vi "Tester.vi"() -> ()   [LabVIEW 2012]
uses:
  <vilib>/Platform/TimedLoop/XDataNode/timing_clust.ctl
  <vilib>/Platform/TimedLoop/XDataNode/nitl_modes.ctl
  <vilib>/Platform/TimedLoop/XDataNode/wakeup.ctl
  <vilib>/rvi/Emulation/niFpgaSctlEmulationRegisterWithScheduler.vi
  <vilib>/rvi/eio/common/nirviEmuTemplateMethod_errors.vi
  <vilib>/rvi/Emulation/niFpgaSctlEmulationScheduler.vi
  <vilib>/rvi/FIFO/Fifo_Resource/nirvififoEmulationSetSize.vi
  <vilib>/rvi/DataTransferAndStorage/Container/Common/niFpgaContainerGetUniqueNameForEmu.vi
  <vilib>/rvi/errors/niFpgaSetErrorForExecOnDevCompSimple.vi
  <vilib>/rvi/eio/common/nirviEmuReportErrorAndStop.vi
  <vilib>/rvi/Emulation/niFpgaSctlEmulationFifoFullMgr.vi
  <vilib>/rvi/Emulation/niFpgaSctlEmulationResourceMgr.vi
  <vilib>/rvi/interface/RandomDataEmulation/nirviRandomDataFPGAFIFO.vi
  <vilib>/rvi/interface/RandomDataEmulation/niFpgaRandomDataHandleErrors.vi
  <vilib>/rvi/Emulation/niFpgaSctlEmulationGlobalWrite.vi
  <vilib>/Platform/TimedLoop/XDataNode/XDataNode.xnode
  <vilib>/eio/EIONode/EIONode.xnode
  <vilib>/rvi/DataTransferAndStorage/Container/XNode/niFpgaContainer.xnode
  <vilib>/rvi/FIFO/Fifo_Resource/nirvififoEmulationClear.vi
  <vilib>/rvi/FIFO/Fifo_Resource/nirvififoEmulationWrite.vi
  <vilib>/rvi/FIFO/Fifo_Resource/nirvififoEmulationRead.vi
  <vilib>/rvi/interface/RandomDataEmulation/nirviRandomDataFpgaReadWriteTemplate.vi
  <vilib>/Platform/TimedLoop/XDataNode/XDNodeRunTimeDep.lvlib
panel:
  out "ToHostArea1LaserRaw FIFO Overflow":bool
  out "ToHostAreas FIFO Overflow":bool
  in  "Laser bitslip":bool
  in  "Laser delay inc":bool
  out "ToHost FIFO Overflow A2Ch1":bool
  in  "Samples per pixel Acq A2":u16=10000 caption="Samples per pixel Acq"
  in  "Samples per pixel Acq A1":u16=10000 caption="Samples per pixel Acq"
  in  "Requested pixels A2":u32=100000 caption="Requested pixels"
  in  "Samples per pixel A2":u16=10000 caption="Samples per pixel"
  out "ToHost FIFO Overflow A1Ch1":bool
  out "Acquiring":bool
  in  "Wait for trigger":bool
  in  "Acquire continuously":bool=TRUE
  in  "Requested pixels A1":u32=100000 caption="Requested pixels"
  in  "Clear Interloop FIFO":bool
  out "Interloop FIFO overflow":bool
  in  "Samples per pixel A1":u16=10000 caption="Samples per pixel"
  in  "Acquire":bool
  out "Interloop FIFO timeout":bool
  in  "Commit":bool
  out "Xpoint_Switch_Ready":bool
  in  "Xpoint_Switch_Write":bool
  in  "Clock Source":u8(ring)=3 items=["Tristate"=0, "Sync Clock (PXIe only)"=2, "Adapter Module Onboard Clock"=3, "Strobe from Crosspoint Switch"=4, "Strobe Bypass"=5]
  in  "Onboard_Clock_Write":bool
  in  "Onboard_Clock_Write_Data":u16
  out "Onboard_Clock_Ready":bool
  in  "Acq_Reset":bool
  # "6587 IO module configuration"
  # "Tester"
  # "Acquisition control"
  # "Area 1"
  # "Area 2"
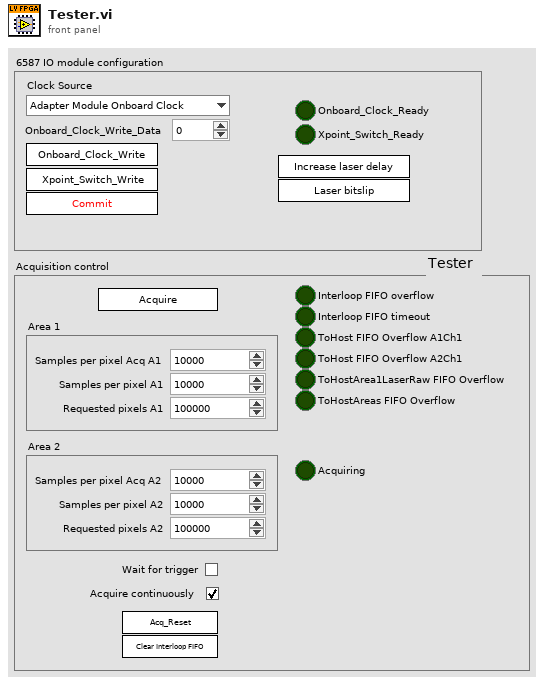
[diagram p1: front panel]
types:
  T1 = typedef "XDNodeRunTimeDep.lvlib/timing_clust.ctl" = cluster{"Expected End [f-1]":u64, "Actual End [f-1]":u64, "Finished Late? [f-1]":bool, "Expected End [i-1]":u64, "Actual End [i-1]":u64, "Finished Late? [i-1]":bool, "Expected Start [i]":u64, "Actual Start [i]":u64, "Expected Start [f]":u64, "Actual Start [f]":u64, "Source Name":string, "Structure Name":string, "Period":i64, "Deadline":i64, "Offset":i64, "Start":i64, "Priority":i32, "Timeout":i32, "Mode":T2, "Wakeup Reason":T3, "Error":errorcluster, "Source Type":string, "Secondary Source Type":string, "Global End Time":u64, "Global Start Time":u64, "Frame Duration":u64, "Iteration Duration":u64, "Assigned CPU":i32, "I/O Scan Engine Mode":u32}
  T2 = typedef "XDNodeRunTimeDep.lvlib/nitl_modes.ctl" = enum32{"No Change", "Process missed periods, maintain original phase", "Discard missed periods, maintain original phase", "Process missed periods, ignore original phase", "Discard missed periods, ignore original phase"}
  T3 = typedef "XDNodeRunTimeDep.lvlib/wakeup.ctl" = enum32{"Normal", "Aborted", "Asynchronous wakeup", "Timing source error", "Timed loop error", "Timeout"}
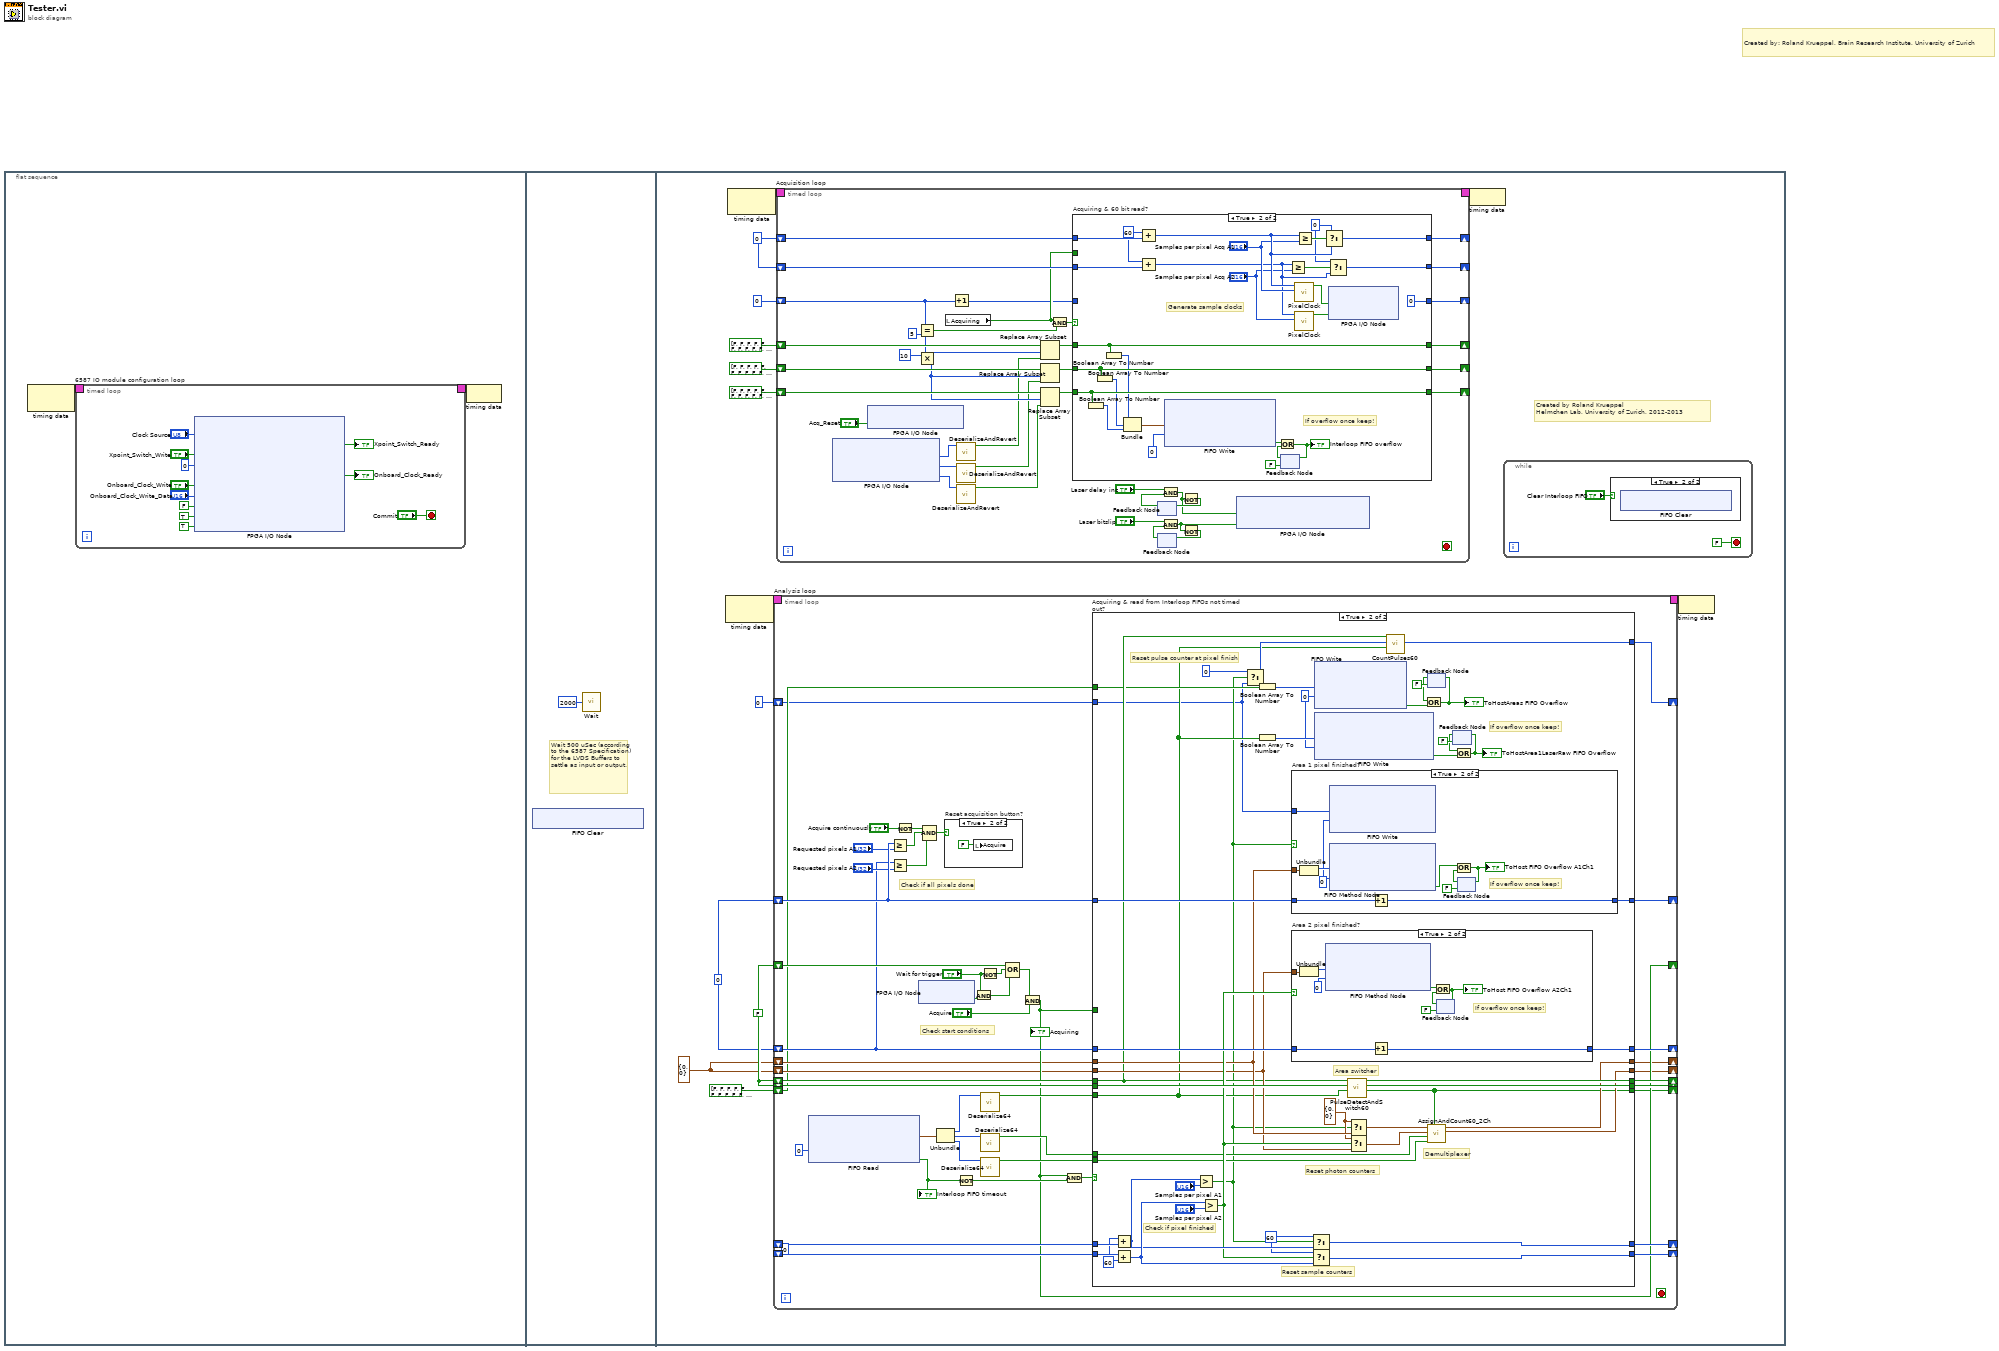
[diagram p0: block diagram]
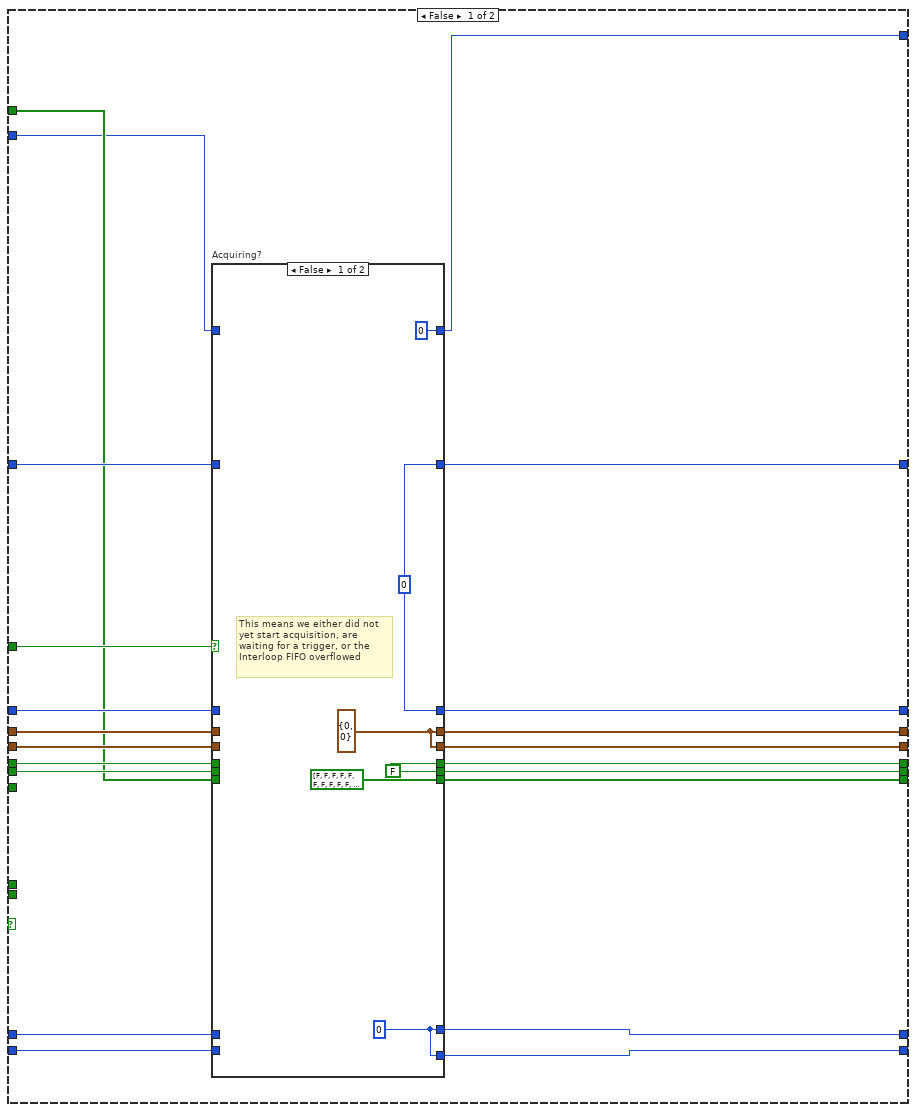
[diagram p4: hidden frame]
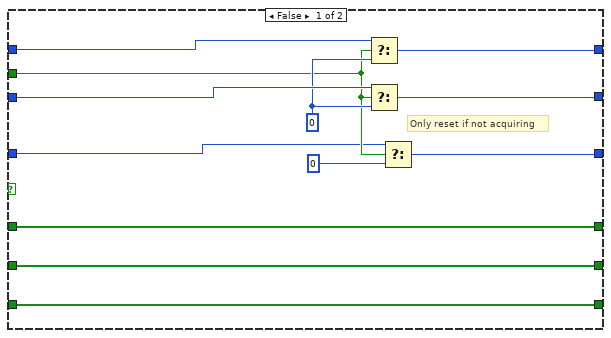
[diagram p8: hidden frame]
diagram:
  # "Created by: Roland Krueppel, Brain Research Institute, University of Zurich"
  n1 = flat-sequence {
    frame #0 {
      n2 = node-c288() -> (w2:T1)  [unwired: 1 in]
      n3 = timed-loop "6587 IO module configuration loop" {
        timing: w2 -> [_]
        timing-out: [_] -> w1
        stop <- "Commit" stop-if-true
        n4 = xnode "FPGA I/O Node"("IO Module\\Acq_IO_Clock_Source"="Clock Source", "IO Module\\Xpoint_Switch_Write"="Xpoint_Switch_Write", "IO Module\\LVDS_Data_Dir"=u16 0 ("IO Module\\LVDS_Data_Dir"), "IO Module\\Onboard_Clock_Write"="Onboard_Clock_Write", "IO Module\\Onboard_Clock_Write_Data"="Onboard_Clock_Write_Data", "IO Module\\SE_PFI0_WE"=FALSE ("IO Module\\SE_PFI0_WE"), "IO Module\\SE_PFI1_WE"=TRUE ("IO Module\\SE_PFI1_WE"), "IO Module\\SE_PFI2_WE"=TRUE ("IO Module\\SE_PFI2_WE")) -> ("IO Module\\Xpoint_Switch_Ready"=→"Xpoint_Switch_Ready":bool, "IO Module\\Onboard_Clock_Ready"=→"Onboard_Clock_Ready":bool)  [unwired: 10 in, 10 out]
      }
      n5 = node-c288(w1) -> ()
    }
    frame #1 {
      # "Wait 500 uSec (according to the 6587 Specification) for the LVDS Buffers to settle as input or output."
      n6 = xnode "FIFO Clear"() -> ()  [unwired: 1 in, 1 out]
      n7 = call "Wait"("Count(uSec)"=u32 2000) -> ()  [unwired: 1 out]
    }
    frame #2 {
      w21 = cluster{u16, u16} {0, 0} ("output cluster")
      w22 = u16 0
      w23 = u32 0 ("Cycle counter out")
      w24 = u16 0
      w25 = FALSE ("Last laser bit out")
      # "Created by Roland Krueppel\nHelmchen Lab, University of Zurich, 2012-2013"
      n8 = node-c288() -> (w31:T1)  [unwired: 1 in]
      n9 = node-c288() -> (w33:T1)  [unwired: 1 in]
      n10 = timed-loop "Analysis loop" {
        timing: w31 -> [_]
        timing-out: [_] -> w30
        shift-right: [w78] -> _
        shift-left: w25 -> [w81]
        shift-right: [w80] -> _
        shift-left: w25 -> [w79]
        shift-right: [w54] -> _
        shift-left: w24 -> [w77]
        shift-right: [w52] -> _
        shift-left: w23 -> [w76]
        shift-right: [w50] -> _
        shift-left: w25 -> [w65]
        shift-right: [w53] -> _
        shift-left: w24 -> [w60]
        shift-right: [w51] -> _
        shift-left: w23 -> [w58]
        shift-right: [w41] -> _
        shift-left: w21 -> [w43]
        shift-right: [w40] -> _
        shift-left: w21 -> [w42]
        shift-right: [w39] -> _
        shift-left: bool[] [FALSE, FALSE, FALSE, FALSE, FALSE, FALSE, FALSE, FALSE, FALSE, FALSE, FALSE, FALSE, FALSE, FALSE, FALSE, FALSE, FALSE, FALSE, FALSE, FALSE, FALSE, FALSE, FALSE, FALSE, FALSE, FALSE, FALSE, FALSE, FALSE, FALSE, FALSE, FALSE, FALSE, FALSE, FALSE, FALSE, FALSE, FALSE, FALSE, FALSE, FALSE, FALSE, FALSE, FALSE, FALSE, FALSE, FALSE, FALSE, FALSE, FALSE, FALSE, FALSE, FALSE, FALSE, FALSE, FALSE, FALSE, FALSE, FALSE, FALSE] ("Area bits out") -> [w38]
        shift-right: [w37] -> _
        shift-left: u16 0 ("New pulse count") -> [w36]
        stop <- _ stop-if-true
        # "Check start conditions"
        # "Check if all pixels done"
        n11 = xnode ("FIFO Read")("Timeout"=0) -> ("Element"=w47:cluster{"Laser":u64, "Ch0":u64, "Ch1":u64}, "Timed Out?"=w48:bool)  [unwired: 1 in, 1 out]
        "Interloop FIFO timeout" <- w48
        n12 = Greater Or Equal?(x=w76, y="Requested pixels A1") -> (x >= y?=w56:bool)
        n13 = Greater Or Equal?(x=w58, y="Requested pixels A2") -> (x >= y?=w55:bool)
        n14 = Not(x="Acquire continuously") -> (.not. x?=w57:bool)
        n15 = xnode "FPGA I/O Node"() -> ("TriggerIn"=w71:bool)  [unwired: 1 in, 1 out]
        n16 = Compound Arithmetic op=AND(w57, w56, w55) -> (w73:bool)
        n17 = Unbundle(w47) -> ("Laser"=w46:u64, "Ch0"=w45:u64, "Ch1"=w44:u64)
        n18 = case "Reset acquisition button?" shown="True" w73 {
          frame False {
          }
          frame True {
            n19 = local write "Acquire"(FALSE ("Acquire")) -> ()
          }
        }
        n20 = Not(x=w48) -> (.not. x?=w66:bool)
        n21 = And(x="Wait for trigger", y=w71) -> (x .and. y?=w68:bool)
        n22 = call "Deserialize64.vi"("U64 input"=w46) -> ("60bit output"=w63:bool[])  [unwired: 10 in]
        n23 = call "Deserialize64.vi"("U64 input"=w45) -> ("60bit output"=w62:bool[])  [unwired: 10 in]
        n24 = call "Deserialize64.vi"("U64 input"=w44) -> ("60bit output"=w61:bool[])  [unwired: 10 in]
        n25 = Not(x="Wait for trigger") -> (.not. x?=w69:bool)
        n26 = Compound Arithmetic op=OR(w65, w69, w68) -> (w67:bool)
        n27 = And(x=w67, y="Acquire") -> (x .and. y?=w50:bool)
        "Acquiring" <- w50
        n28 = And(x=w50, y=w66) -> (x .and. y?=w64:bool)
        n29 = case "Acquiring & read from Interloop FIFOs not timed out?" shown="True" w64 {
          tunnel: w81 -> [w98 w152]
          tunnel: w43 -> [w102 w148]
          tunnel: [w97 w151] -> w80
          tunnel: w79 -> [w99 w138]
          tunnel: [w96 w150] -> w78
          tunnel: w77 -> [w101 w166]
          tunnel: w76 -> [w100 w162]
          tunnel: w63 -> [_ w131]
          tunnel: w62 -> [_ w144]
          tunnel: w50 -> [w103 _]
          tunnel: w61 -> [_ w143]
          tunnel: w60 -> [w90 w164]
          tunnel: w58 -> [w93 w161]
          tunnel: [w91 w154] -> w54
          tunnel: [w89 w156] -> w53
          tunnel: [w95 w141] -> w41
          tunnel: [w94 w159] -> w52
          tunnel: [w92 w160] -> w51
          tunnel: w42 -> [w88 w146]
          tunnel: [w87 w140] -> w40
          tunnel: [w85 w139] -> w39
          tunnel: w38 -> [w86 w133]
          tunnel: [w83 w137] -> w37
          tunnel: w36 -> [w84 w128]
          frame False {
            n30 = case "Acquiring?" shown="False" w103 {
              tunnel: w102 -> [_ w117]
              tunnel: w101 -> [_ w114]
              tunnel: w100 -> [_ w116]
              tunnel: w99 -> [_ w119]
              tunnel: w98 -> [_ w118]
              tunnel: [w109 w119] -> w97
              tunnel: [w109 w118] -> w96
              tunnel: [w107 w117] -> w95
              tunnel: [w108 w116] -> w94
              tunnel: w93 -> [_ w115]
              tunnel: [w108 w115] -> w92
              tunnel: [w106 w114] -> w91
              tunnel: [w106 w113] -> w89
              tunnel: w90 -> [_ w113]
              tunnel: w88 -> [_ w112]
              tunnel: [w107 w112] -> w87
              tunnel: w86 -> [_ w111]
              tunnel: [bool[] [FALSE, FALSE, FALSE, FALSE, FALSE, FALSE, FALSE, FALSE, FALSE, FALSE, FALSE, FALSE, FALSE, FALSE, FALSE, FALSE, FALSE, FALSE, FALSE, FALSE, FALSE, FALSE, FALSE, FALSE, FALSE, FALSE, FALSE, FALSE, FALSE, FALSE, FALSE, FALSE, FALSE, FALSE, FALSE, FALSE, FALSE, FALSE, FALSE, FALSE, FALSE, FALSE, FALSE, FALSE, FALSE, FALSE, FALSE, FALSE, FALSE, FALSE, FALSE, FALSE, FALSE, FALSE, FALSE, FALSE, FALSE, FALSE, FALSE, FALSE] ("Area bits out") w111] -> w85
              tunnel: w84 -> [_ w110]
              tunnel: [u16 0 ("New pulse count") w110] -> w83
              frame False {
                w107 = cluster{u16, u16} {0, 0} ("output cluster")
                w108 = u32 0 ("Cycle counter out")
                w106 = u16 0
                w109 = FALSE ("Last laser bit out")
                # "This means we either did not\nyet start acquisition, are\nwaiting for a trigger, or the\nInterloop FIFO overflowed"
              }
              frame True {
                # "This means we are\nreading faster here\nthan acquiring in\nAcquisition loop\n-> keep all values"
              }
            }
          }
          frame True {
            w130 = 0 ("Timeout")
            w142 = cluster{u16, u16} {0, 0} ("t")
            w153 = u16 60 ("t")
            w163 = u16 60
            # "If overflow once keep!"
            # "Reset pulse counter at pixel finish"
            # "Demultiplexer"
            # "Reset photon counters"
            # "Area switcher"
            # "Check if pixel finished"
            # "Reset sample counters"
            n31 = Add(x=w163, y=w166) -> (x+y=w155:u16)
            n32 = Add(x=w164, y=w163) -> (x+y=w157:u16)
            n33 = Greater?(x=w155, y="Samples per pixel A1") -> (0:w129:bool)
            n34 = Greater?(x=w157, y="Samples per pixel A2") -> (0:w149:bool)
            n35 = Select(t=u16 0, s=w129, f=w128) -> (s? t:f=w136:u16)
            n36 = Boolean Array To Number(Boolean array=w133) -> (number=w134:u64)
            n37 = Boolean Array To Number(Boolean array=w131) -> (number=w132:u64)
            n38 = case "Area 1 pixel finished?" shown="True" w129 {
              tunnel: w148 -> [_ w185]
              tunnel: w162 -> [w177 w187]
              tunnel: [w177 w186] -> w159
              tunnel: w128 -> [_ w182]
              frame False {
              }
              frame True {
                w183 = 0 ("Timeout")
                # "If overflow once keep!"
                n39 = Unbundle(w185) -> (w184:u16)  [unwired: 1 out]
                n40 = xnode ("FIFO Write")("Element"=w182, "Timeout"=w183) -> ()  [unwired: 1 in, 2 out]
                n41 = xnode ("FIFO Method Node")("Element"=w184, "Timeout"=w183) -> ("Timed Out?"=w180:bool)  [unwired: 1 in, 1 out]
                n42 = Increment(x=w187) -> (x+1=w186:u32)
                n43 = feedback #1(FALSE) -> (w179:bool)
                n44 = Or(x=w180, y=w179) -> (x .or. y?=w178:bool)
                "ToHost FIFO Overflow A1Ch1" <- w178
                n45 = feedback-in #1(w178) -> ()
              }
            }
            n46 = case "Area 2 pixel finished?" shown="True" w149 {
              tunnel: w161 -> [w167 w175]
              tunnel: [w167 w174] -> w160
              tunnel: w146 -> [_ w173]
              frame False {
              }
              frame True {
                # "If overflow once keep!"
                n47 = Unbundle(w173) -> (w172:u16)  [unwired: 1 out]
                n48 = xnode ("FIFO Method Node")("Element"=w172, "Timeout"=0) -> ("Timed Out?"=w170:bool)  [unwired: 1 in, 1 out]
                n49 = Increment(x=w175) -> (x+1=w174:u32)
                n50 = feedback #2(FALSE) -> (w169:bool)
                n51 = Or(x=w170, y=w169) -> (x .or. y?=w168:bool)
                "ToHost FIFO Overflow A2Ch1" <- w168
                n52 = feedback-in #2(w168) -> ()
              }
            }
            n53 = Select(t=w153, s=w129, f=w155) -> (s? t:f=w154:u16)
            n54 = Select(t=w153, s=w149, f=w157) -> (s? t:f=w156:u16)
            n55 = xnode ("FIFO Write")("Element"=w134, "Timeout"=w130) -> ("Timed Out?"=w126:bool)  [unwired: 1 in, 1 out]
            n56 = xnode ("FIFO Write")("Element"=w132, "Timeout"=w130) -> ("Timed Out?"=w121:bool)  [unwired: 1 in, 1 out]
            n57 = call "PulseDetectAndSwitch60.vi"("Laser bits in"=w131, "Last area"=w152, "Last laser bit in"=w138) -> ("Area bits out"=w139:bool[], "New last area out"=w150:bool, "New last laser bit out"=w151:bool)  [unwired: 6 in]
            n58 = Select(t=w142, s=w129, f=w148) -> (s? t:f=w147:cluster{u16, u16})
            n59 = Select(t=w142, s=w149, f=w146) -> (s? t:f=w145:cluster{u16, u16})
            n60 = call "CountPulses60.vi"("60bit input"=w131, "Previous pulse count"=w136, "Last sample"=w138) -> ("New pulse count"=w137:u16)  [unwired: 7 in, 1 out]
            n61 = feedback #3(FALSE) -> (w125:bool)
            n62 = Or(x=w125, y=w126) -> (x .or. y?=w124:bool)
            "ToHostAreas FIFO Overflow" <- w124
            n63 = feedback-in #3(w124) -> ()
            n64 = call "AssignAndCount60_2Ch.vi"("Area bits in"=w139, "PMT bits Ch2 in"=w143, "PMT bits Ch1 in"=w144, "Photon counters area 2 in"=w145, "Photon counters area 1 in"=w147) -> ("Photon counters area 2 out"=w140:cluster{u16, u16}, "Photon counters area 1 out"=w141:cluster{u16, u16})  [unwired: 5 in]
            n65 = feedback #4(FALSE) -> (w122:bool)
            n66 = Or(x=w122, y=w121) -> (x .or. y?=w120:bool)
            "ToHostArea1LaserRaw FIFO Overflow" <- w120
            n67 = feedback-in #4(w120) -> ()
          }
        }
      }
      n68 = timed-loop "Acquisition loop" {
        timing: w33 -> [_]
        timing-out: [_] -> w32
        shift-right: [w219] -> _
        shift-left: bool[] [FALSE, FALSE, FALSE, FALSE, FALSE, FALSE, FALSE, FALSE, FALSE, FALSE, FALSE, FALSE, FALSE, FALSE, FALSE, FALSE, FALSE, FALSE, FALSE, FALSE, FALSE, FALSE, FALSE, FALSE, FALSE, FALSE, FALSE, FALSE, FALSE, FALSE, FALSE, FALSE, FALSE, FALSE, FALSE, FALSE, FALSE, FALSE, FALSE, FALSE, FALSE, FALSE, FALSE, FALSE, FALSE, FALSE, FALSE, FALSE, FALSE, FALSE, FALSE, FALSE, FALSE, FALSE, FALSE, FALSE, FALSE, FALSE, FALSE, FALSE, FALSE, FALSE, FALSE, FALSE] ("Boolean array") -> [w227]
        shift-right: [w218] -> _
        shift-left: bool[] [FALSE, FALSE, FALSE, FALSE, FALSE, FALSE, FALSE, FALSE, FALSE, FALSE, FALSE, FALSE, FALSE, FALSE, FALSE, FALSE, FALSE, FALSE, FALSE, FALSE, FALSE, FALSE, FALSE, FALSE, FALSE, FALSE, FALSE, FALSE, FALSE, FALSE, FALSE, FALSE, FALSE, FALSE, FALSE, FALSE, FALSE, FALSE, FALSE, FALSE, FALSE, FALSE, FALSE, FALSE, FALSE, FALSE, FALSE, FALSE, FALSE, FALSE, FALSE, FALSE, FALSE, FALSE, FALSE, FALSE, FALSE, FALSE, FALSE, FALSE, FALSE, FALSE, FALSE, FALSE] ("Boolean array") -> [w226]
        shift-right: [w217] -> _
        shift-left: 0 -> [w216]
        shift-right: [w212] -> _
        shift-left: bool[] [FALSE, FALSE, FALSE, FALSE, FALSE, FALSE, FALSE, FALSE, FALSE, FALSE, FALSE, FALSE, FALSE, FALSE, FALSE, FALSE, FALSE, FALSE, FALSE, FALSE, FALSE, FALSE, FALSE, FALSE, FALSE, FALSE, FALSE, FALSE, FALSE, FALSE, FALSE, FALSE, FALSE, FALSE, FALSE, FALSE, FALSE, FALSE, FALSE, FALSE, FALSE, FALSE, FALSE, FALSE, FALSE, FALSE, FALSE, FALSE, FALSE, FALSE, FALSE, FALSE, FALSE, FALSE, FALSE, FALSE, FALSE, FALSE, FALSE, FALSE, FALSE, FALSE, FALSE, FALSE] ("Boolean array") -> [w215]
        shift-right: [w210] -> _
        shift-left: w22 -> [w211]
        shift-right: [w208] -> _
        shift-left: w22 -> [w209]
        stop <- _ stop-if-true
        n69 = xnode "FPGA I/O Node"() -> ("IO Module\\LVDS_Ch0_Rd"=w205:u16, "IO Module\\LVDS_Ch1_Rd"=w203:u16, "IO Module\\LVDS_Ch2_Rd"=w201:u16)  [unwired: 3 in, 3 out]
        n70 = xnode "FPGA I/O Node"("IO Module\\Acq_Reset"="Acq_Reset") -> ()  [unwired: 1 in, 1 out]
        n71 = Equal?(x=w216, y=5) -> (x = y?=w223:bool)
        n72 = Multiply(x=10 ("y"), y=w216) -> (x*y=w214:i32)
        n73 = local read "Acquiring"() -> (w207:bool)
        n74 = Increment(x=w216) -> (x+1=w206:i32)
        n75 = call "DeserializeAndRevert.vi"("U16 input"=w205) -> ("10bit output"=w204:bool[])  [unwired: 10 in]
        n76 = call "DeserializeAndRevert.vi"("U16 input"=w203) -> ("10bit output"=w202:bool[])  [unwired: 10 in]
        n77 = call "DeserializeAndRevert.vi"("U16 input"=w201) -> ("10bit output"=w200:bool[])  [unwired: 10 in]
        n78 = Replace Array Subset(array=w227, new element=w204, index=w214) -> (w221:bool[])
        n79 = Replace Array Subset(array=w226, new element=w202, index=w214) -> (w220:bool[])
        n80 = Replace Array Subset(array=w215, new element=w200, index=w214) -> (w213:bool[])
        n81 = And(x=w207, y=w223) -> (x .and. y?=w222:bool)
        n82 = case "Acquiring & 60 bit read?" shown="True" w222 {
          tunnel: w221 -> [w240 w264]
          tunnel: w220 -> [w239 w266]
          tunnel: [w240 w264] -> w219
          tunnel: [w239 w266] -> w218
          tunnel: [w230 0] -> w217
          tunnel: w206 -> [w231 _]
          tunnel: w213 -> [w238 w265]
          tunnel: [w238 w265] -> w212
          tunnel: w211 -> [w237 w263]
          tunnel: [w236 w261] -> w210
          tunnel: w209 -> [w235 w257]
          tunnel: [w234 w253] -> w208
          tunnel: w207 -> [w232 _]
          frame False {
            w233 = u16 0 ("f")
            # "Only reset if not acquiring"
            n83 = Select(t=w237, s=w232, f=w233) -> (s? t:f=w236:u16)
            n84 = Select(t=w235, s=w232, f=w233) -> (s? t:f=w234:u16)
            n85 = Select(t=w231, s=w232, f=0) -> (s? t:f=w230:i32)
          }
          frame True {
            w254 = u16 0 ("t")
            w256 = u16 60 ("x")
            # "If overflow once keep!"
            # "Generate sample clocks"
            n86 = Boolean Array To Number(Boolean array=w265) -> (number=w247:u64)
            n87 = Boolean Array To Number(Boolean array=w266) -> (number=w248:u64)
            n88 = Boolean Array To Number(Boolean array=w264) -> (number=w249:u64)
            n89 = Bundle(w249, w248, w247) -> (w246:cluster{u64, u64, u64})  [unwired: 1 in]
            n90 = Add(x=w256, y=w263) -> (x+y=w260:u16)
            n91 = Add(x=w256, y=w257) -> (x+y=w252:u16)
            n92 = xnode ("FIFO Write")("Element"=w246, "Timeout"=0) -> ("Timed Out?"=w242:bool)  [unwired: 1 in, 1 out]
            n93 = feedback #5(FALSE) -> (w244:bool)
            n94 = Or(x=w242, y=w244) -> (x .or. y?=w241:bool)
            "Interloop FIFO overflow" <- w241
            n95 = feedback-in #5(w241) -> ()
            n96 = Greater Or Equal?(x=w252, y="Samples per pixel Acq A2") -> (x >= y?=w255:bool)
            n97 = call "PixelClock.vi"("Samples per pixel"="Samples per pixel Acq A1", "Sample counter"=w260) -> ("Pixel clock"=w258:bool)  [unwired: 9 in]
            n98 = call "PixelClock.vi"("Samples per pixel"="Samples per pixel Acq A2", "Sample counter"=w252) -> ("Pixel clock"=w250:bool)  [unwired: 9 in]
            n99 = Greater Or Equal?(x=w260, y="Samples per pixel Acq A1") -> (x >= y?=w262:bool)
            n100 = Select(t=w254, s=w262, f=w260) -> (s? t:f=w261:u16)
            n101 = Select(t=w254, s=w255, f=w252) -> (s? t:f=w253:u16)
            n102 = xnode "FPGA I/O Node"("Pixel clock A1"=w258, "Pixel clock A2"=w250) -> ()  [unwired: 2 in, 2 out]
          }
        }
        n103 = feedback #6() -> (w198:bool)  [unwired: 1 in]
        n104 = feedback #7() -> (w193:bool)  [unwired: 1 in]
        n105 = And(x="Laser delay inc", y=w198) -> (x .and. y?=w196:bool)
        n106 = And(x="Laser bitslip", y=w193) -> (x .and. y?=w192:bool)
        n107 = Not(x=w196) -> (.not. x?=w197:bool)
        n108 = feedback-in #6(w197) -> ()
        n109 = Not(x=w192) -> (.not. x?=w195:bool)
        n110 = feedback-in #7(w195) -> ()
        n111 = xnode "FPGA I/O Node"("IO Module\\Ch0_Idelay_Increment"=w196, "IO Module\\Ch0_Bitslip"=w192) -> ()  [unwired: 2 in, 2 out]
      }
      n112 = node-c288(w32) -> ()
      n113 = while {
        stop <- FALSE stop-if-true
        n114 = case shown="True" "Clear Interloop FIFO" {
          frame False {
          }
          frame True {
            n115 = xnode ("FIFO Clear")() -> ()  [unwired: 1 in, 1 out]
          }
        }
      }
      n116 = node-c288(w30) -> ()
    }
  }
